vi "ReadFromTextFile_v2.vi"(6 "Display Data":bool, 7 "Convert Phase to Radians":bool, 8 "Convert Amplitude to dB":bool, 9 "Skip First N Lines":i32=48, 10 "name or relative path":path=path "C:/Users/LAV-UFSC/OneDrive - UFSC/Documents/LAV - TCC/Dados-Experimentos/25-04/frf_2.txt") -> (0 "Phase":dbl[][](array[numeric]), 1 "Magnitude":dbl[][](array[numeric]), 2 "Phase":cluster{dbl[], dbl[]}, 3 "Magnitude":cluster{dbl[], dbl[]})   [LabVIEW 2022 SP3]
uses:
  <vilib>/Utility/file.llb/Read Delimited Spreadsheet (DBL).vi
panel:
  in  "Output Type":bool
  out "Phase":cluster{"Array":dbl[], "Array":dbl[]}(graph) caption="Amplitude [Hz]"
  out "Magnitude":cluster{"Array":dbl[], "Array":dbl[]}(graph) caption="Amplitude [Hz]"
  out "number of rows":i32
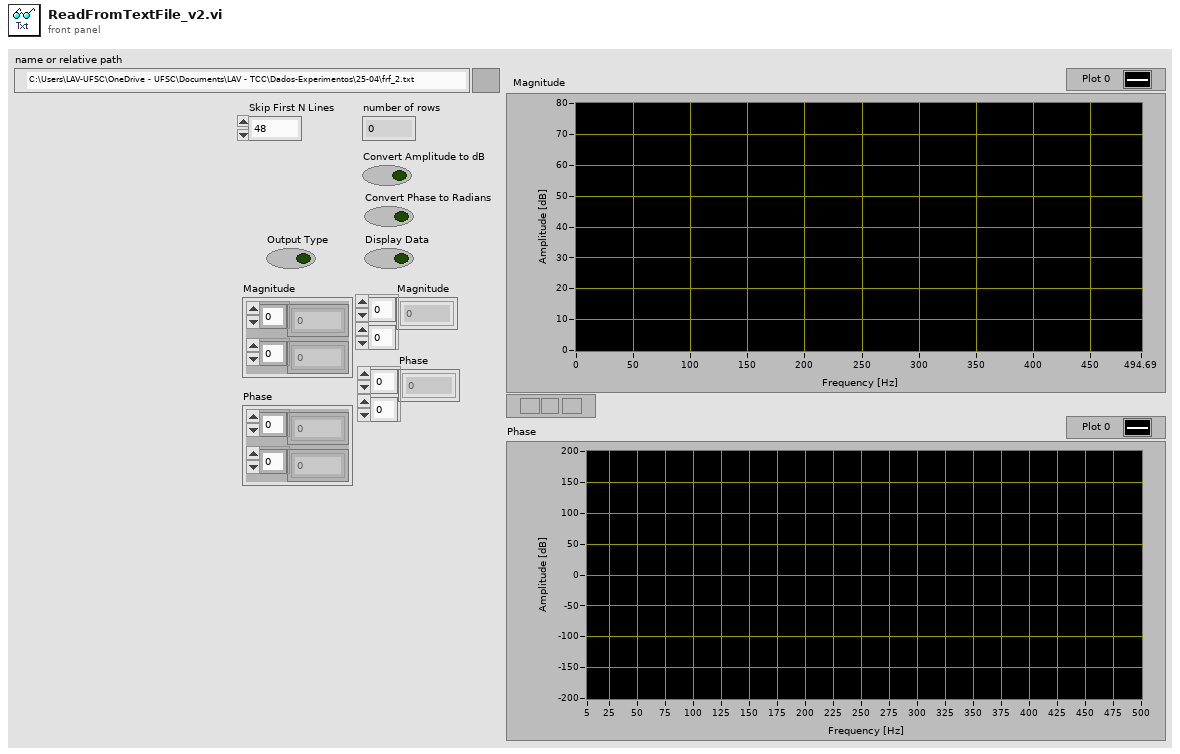
[diagram p1: front panel]
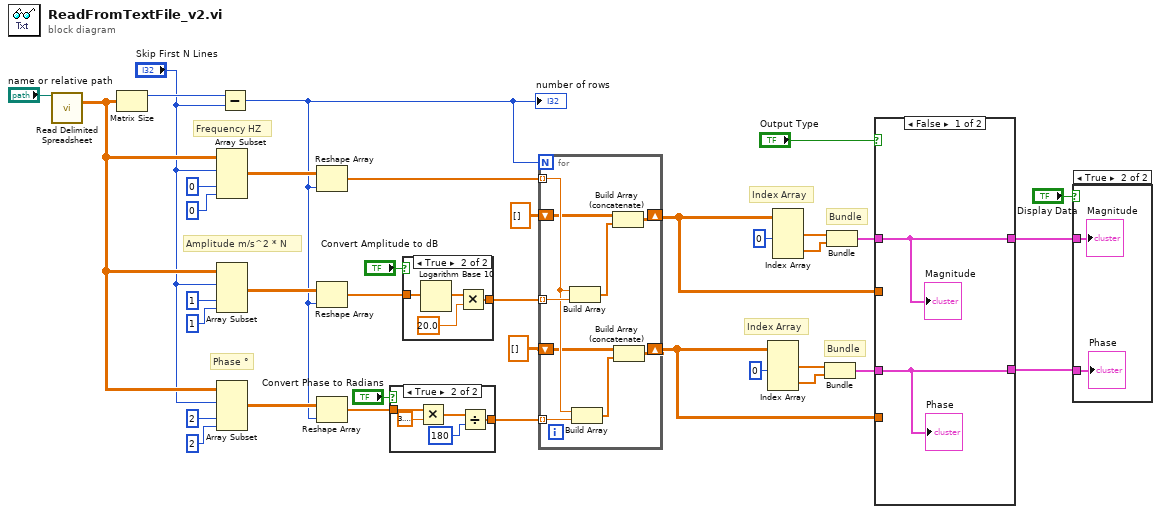
[diagram p0: block diagram]
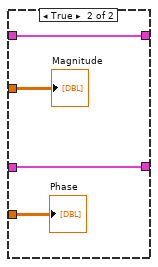
[diagram p2: hidden frame]
diagram:
  # "Index Array"
  # "Bundle"
  # "Index Array"
  # "Bundle"
  # "Phase °"
  # "Amplitude m/s^2 * N"
  # "Frequency HZ"
  n1 = call-poly <vilib>:"Read Delimited Spreadsheet.vi"("file path (dialog if empty)"="name or relative path") -> ("all rows"=w28:dbl[][])  [unwired: 9 in, 5 out]
  n2 = Matrix Size(0:w28) -> (1:w16:i32)  [unwired: 1 out]
  n3 = Array Subset(array=w28, index (row)="Skip First N Lines", index (col)=0 ("column 1"), length (col)=0 ("column N")) -> (w30:dbl[][])  [unwired: 1 in]
  n4 = Array Subset(array=w28, index (row)="Skip First N Lines", index (col)=1 ("column 1"), length (col)=1 ("column N")) -> (w29:dbl[][])  [unwired: 1 in]
  n5 = Array Subset(array=w28, index (row)="Skip First N Lines", index (col)=2 ("column 1"), length (col)=2 ("column N")) -> (w17:dbl[][])  [unwired: 1 in]
  n6 = Subtract(x=w16, y="Skip First N Lines") -> (x-y=w14:i32)
  "number of rows" <- w14
  n7 = Reshape Array(w30, w14) -> (w13:dbl[])
  n8 = Reshape Array(w29, w14) -> (w12:dbl[])
  n9 = Reshape Array(w17, w14) -> (w10:dbl[])
  n10 = case shown="True" "Convert Phase to Radians" {
    tunnel: w10 -> [w38 w42]
    tunnel: [w38 w39] -> w9
    frame False {
    }
    frame True {
      n11 = Multiply(x=w42, y=3.141592653589793) -> (x*y=w43:dbl[])
      n12 = Divide(x=w43, y=180) -> (x/y=w39:dbl[])
    }
  }
  n13 = case shown="True" "Convert Amplitude to dB" {
    tunnel: [w44 w46] -> w23
    tunnel: w12 -> [w44 w45]
    frame False {
    }
    frame True {
      n14 = Logarithm Base 10(1:w45) -> (0:w47:dbl[])
      n15 = Multiply(x=w47, y=20.0) -> (x*y=w46:dbl[])
    }
  }
  n16 = for {
    N: w14 -> [_]
    tunnel: w13 -> [w55] mode=indexing
    tunnel: w23 -> [w56] mode=indexing
    tunnel: w9 -> [w57] mode=indexing
    shift-right: [w52] -> w6
    shift-left: dbl[][] [] -> [w54]
    shift-right: [w51] -> w18
    shift-left: dbl[][] [] -> [w50]
    n17 = Build Array(w55, w56) -> (w53:dbl[])
    n18 = Build Array(w55, w57) -> (w49:dbl[])
    n19 = Build Array (concatenate)(w54, w53) -> (w52:dbl[][])
    n20 = Build Array (concatenate)(w50, w49) -> (w51:dbl[][])
  }
  n21 = Index Array(array=w18, index (col) #1=0 ("disabled index (col)")) -> (element #1=w19:dbl[], element #2=w20:dbl[])  [unwired: 3 in]
  n22 = Index Array(array=w6, index (col) #1=0 ("disabled index (col)")) -> (element #1=w24:dbl[], element #2=w25:dbl[])  [unwired: 3 in]
  n23 = Bundle(w19, w20) -> (w4:cluster{dbl[], dbl[]})  [unwired: 1 in]
  n24 = Bundle(w24, w25) -> (w2:cluster{dbl[], dbl[]})  [unwired: 1 in]
  n25 = case shown="False" "Output Type" {
    tunnel: w18 -> [_ w63]
    tunnel: w6 -> [_ w62]
    tunnel: w4 -> [w58 w61]
    tunnel: [w58 w61] -> w3
    tunnel: w2 -> [w59 w60]
    tunnel: [w59 w60] -> w1
    frame False {
      "Magnitude" <- w59
      "Phase" <- w58
    }
    frame True {
      "Phase" <- w63
      "Magnitude" <- w62
    }
  }
  n26 = case shown="True" "Display Data" {
    tunnel: w1 -> [_ w65]
    tunnel: w3 -> [_ w64]
    frame False {
    }
    frame True {
      "Magnitude" <- w65
      "Phase" <- w64
    }
  }
